vi "Tracker_Settings.vi"(0 "input cluster":T3, 2 "Directory Exists?":refnum<vi>) -> (1 "output cluster":T4)   [LabVIEW 2015]
uses:
  <vilib>/vision/Avi1.llb/AviRefnum.ctl
  <vilib>/userdefined/High Color/IMAQdx.ctl
panel:
  out "custom 2 timing array":dbl[](array[numeric])
  out "custom timing array":dbl[](array[numeric])
  out "puff timing array":dbl[](array[numeric])
  out "tap timing array":dbl[](array[numeric])
  out "AFG Settings":dbl[][](array[numeric])
  out "settings value cluster":T5
  out "Output  ROI Array":dbl[][](array[numeric])
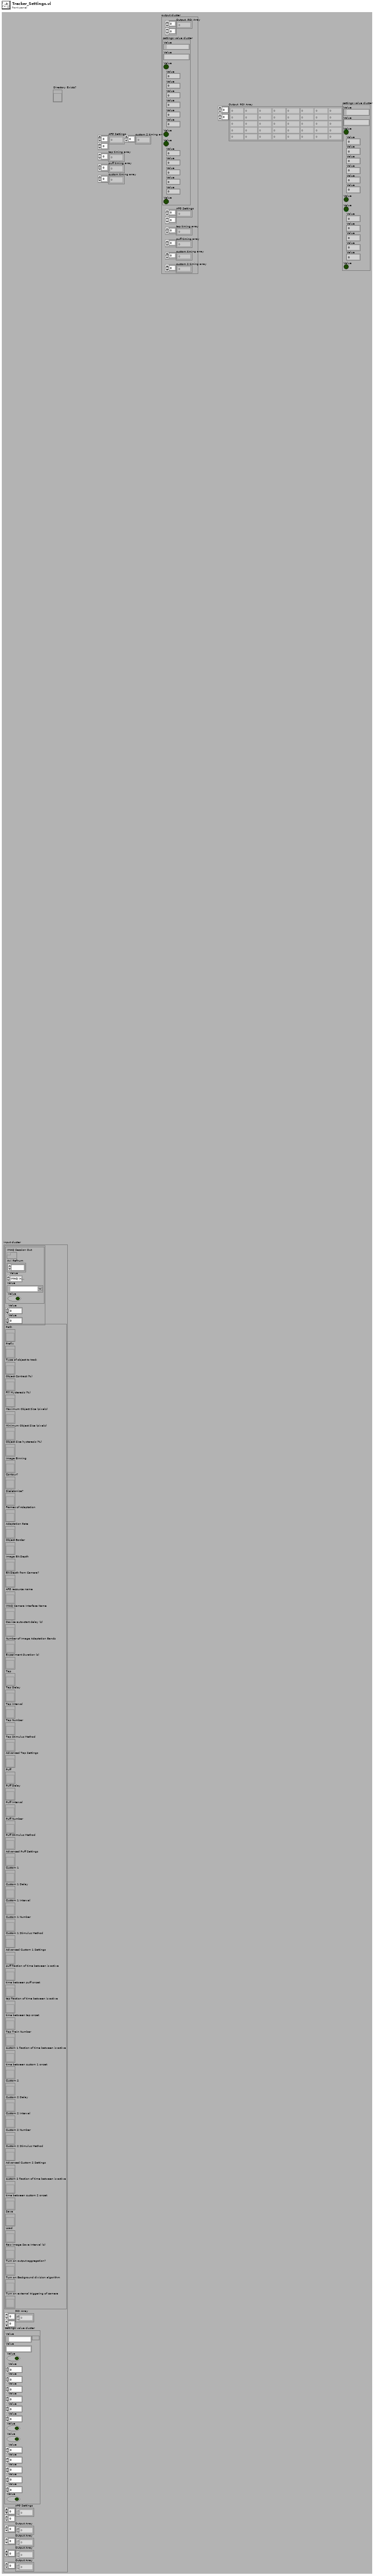
[diagram p1: front panel]
types:
  T1 = typedef "AviRefnum.ctl" = refnum<k1>
  T2 = typedef "IMAQdx.ctl" = refnum<k21>
  T3 = cluster{cluster{cluster{"IMAQ Session Out":refnum<k11>, "Avi Refnum":T1, "Value":enum32{"IMAQ interface", "IMAQdx interface", "AVI file"}, "Value":T2, "Value":bool}, "Value":i32, "Value":i32}, cluster{"Path":refnum<vi>, "Prefix":refnum<vi>, "Type of object to track":refnum<vi>, "Object Contrast (%)":refnum<vi>, "Fill Hysteresis (%)":refnum<vi>, "Maximum Object Size (pixels)":refnum<vi>, "Minimum Object Size (pixels)":refnum<vi>, "Object Size hysteresis (%)":refnum<vi>, "Image Binning":refnum<vi>, "Contour?":refnum<vi>, "Skeletonize?":refnum<vi>, "Frames of Adaptation":refnum<vi>, "Adaptation Rate":refnum<vi>, "Object Border":refnum<vi>, "Image Bit Depth":refnum<vi>, "Bit Depth from Camera?":refnum<vi>, "AFG resource name":refnum<vi>, "IMAQ Camera Interface Name":refnum<vi>, "Device auto-start delay (s)":refnum<vi>, "Number of Image Adaptation Bands":refnum<vi>, "Experiment Duration (s)":refnum<vi>, "Tap":refnum<vi>, "Tap Delay":refnum<vi>, "Tap Interval":refnum<vi>, "Tap Number":refnum<vi>, "Tap Stimulus Method":refnum<vi>, "Advanced Tap Settings":refnum<vi>, "Puff":refnum<vi>, "Puff Delay":refnum<vi>, "Puff Interval":refnum<vi>, "Puff Number":refnum<vi>, "Puff Stimulus Method":refnum<vi>, "Advanced Puff Settings":refnum<vi>, "Custom 1":refnum<vi>, "Custom 1 Delay":refnum<vi>, "Custom 1 Interval":refnum<vi>, "Custom 1 Number":refnum<vi>, "Custom 1 Stimulus Method":refnum<vi>, "Advanced Custom 1 Settings":refnum<vi>, "puff fraction of time between is active":refnum<vi>, "time between puff onset":refnum<vi>, "tap fraction of time between is active":refnum<vi>, "time between tap onset":refnum<vi>, "Tap Train Number":refnum<vi>, "custom 1 fraction of time between is active":refnum<vi>, "time between custom 1 onset":refnum<vi>, "Custom 2":refnum<vi>, "Custom 2 Delay":refnum<vi>, "Custom 2 Interval":refnum<vi>, "Custom 2 Number":refnum<vi>, "Custom 2 Stimulus Method":refnum<vi>, "Advanced Custom 2 Settings":refnum<vi>, "custom 2 fraction of time between is active":refnum<vi>, "time between custom 2 onset":refnum<vi>, "Save":refnum<vi>, "Load":refnum<vi>, "Raw Image Save Interval (s)":refnum<vi>, "Turn on output aggregation?":refnum<vi>, "Turn on Background division algorithm":refnum<vi>, "Turn on external triggering of camera":refnum<vi>}, "ROI Array":dbl[][], "settings value cluster":cluster{"Value":path, "Value":string, "Value":bool, "Value":dbl, "Value":dbl, "Value":i32, "Value":i32, "Value":dbl, "Value":u16, "Value":bool, "Value":bool, "Value":i32, "Value":i32, "Value":i32, "Value":u32, "Value":i32, "Value":bool}, "AFG Settings":dbl[][], "Output Array":dbl[], "Output Array":dbl[], "Output Array":dbl[], "Output Array":dbl[]}
  T4 = cluster{"Output  ROI Array":dbl[][], "settings value cluster":cluster{"Value":path, "Value":string, "Value":bool, "Value":dbl, "Value":dbl, "Value":i32, "Value":i32, "Value":dbl, "Value":u16, "Value":bool, "Value":bool, "Value":i32, "Value":i32, "Value":i32, "Value":u32, "Value":i32, "Value":bool}, "AFG Settings":dbl[][], "tap timing array":dbl[], "puff timing array":dbl[], "custom timing array":dbl[], "custom 2 timing array":dbl[]}
  T5 = cluster{"Value":path, "Value":string, "Value":bool, "Value":dbl, "Value":dbl, "Value":i32, "Value":i32, "Value":dbl, "Value":u16, "Value":bool, "Value":bool, "Value":i32, "Value":i32, "Value":i32, "Value":u32, "Value":i32, "Value":bool}
  T6 = cluster{cluster{"IMAQ Session Out":refnum<k11>, "Avi Refnum":T1, "Value":enum32{"IMAQ interface", "IMAQdx interface", "AVI file"}, "Value":T2, "Value":bool}, "Value":i32, "Value":i32}
  T7 = cluster{"Path":refnum<vi>, "Prefix":refnum<vi>, "Type of object to track":refnum<vi>, "Object Contrast (%)":refnum<vi>, "Fill Hysteresis (%)":refnum<vi>, "Maximum Object Size (pixels)":refnum<vi>, "Minimum Object Size (pixels)":refnum<vi>, "Object Size hysteresis (%)":refnum<vi>, "Image Binning":refnum<vi>, "Contour?":refnum<vi>, "Skeletonize?":refnum<vi>, "Frames of Adaptation":refnum<vi>, "Adaptation Rate":refnum<vi>, "Object Border":refnum<vi>, "Image Bit Depth":refnum<vi>, "Bit Depth from Camera?":refnum<vi>, "AFG resource name":refnum<vi>, "IMAQ Camera Interface Name":refnum<vi>, "Device auto-start delay (s)":refnum<vi>, "Number of Image Adaptation Bands":refnum<vi>, "Experiment Duration (s)":refnum<vi>, "Tap":refnum<vi>, "Tap Delay":refnum<vi>, "Tap Interval":refnum<vi>, "Tap Number":refnum<vi>, "Tap Stimulus Method":refnum<vi>, "Advanced Tap Settings":refnum<vi>, "Puff":refnum<vi>, "Puff Delay":refnum<vi>, "Puff Interval":refnum<vi>, "Puff Number":refnum<vi>, "Puff Stimulus Method":refnum<vi>, "Advanced Puff Settings":refnum<vi>, "Custom 1":refnum<vi>, "Custom 1 Delay":refnum<vi>, "Custom 1 Interval":refnum<vi>, "Custom 1 Number":refnum<vi>, "Custom 1 Stimulus Method":refnum<vi>, "Advanced Custom 1 Settings":refnum<vi>, "puff fraction of time between is active":refnum<vi>, "time between puff onset":refnum<vi>, "tap fraction of time between is active":refnum<vi>, "time between tap onset":refnum<vi>, "Tap Train Number":refnum<vi>, "custom 1 fraction of time between is active":refnum<vi>, "time between custom 1 onset":refnum<vi>, "Custom 2":refnum<vi>, "Custom 2 Delay":refnum<vi>, "Custom 2 Interval":refnum<vi>, "Custom 2 Number":refnum<vi>, "Custom 2 Stimulus Method":refnum<vi>, "Advanced Custom 2 Settings":refnum<vi>, "custom 2 fraction of time between is active":refnum<vi>, "time between custom 2 onset":refnum<vi>, "Save":refnum<vi>, "Load":refnum<vi>, "Raw Image Save Interval (s)":refnum<vi>, "Turn on output aggregation?":refnum<vi>, "Turn on Background division algorithm":refnum<vi>, "Turn on external triggering of camera":refnum<vi>}
  T8 = cluster{"IMAQ Session Out":refnum<k11>, "Avi Refnum":T1, "Value":enum32{"IMAQ interface", "IMAQdx interface", "AVI file"}, "Value":T2, "Value":bool}
  T9 = cluster{dbl[][], dbl[][], dbl[], dbl[], dbl[], dbl[]}
  T10 = cluster{cluster{"Path":refnum<vi>, "Prefix":refnum<vi>, "Type of object to track":refnum<vi>, "Object Contrast (%)":refnum<vi>, "Fill Hysteresis (%)":refnum<vi>, "Maximum Object Size (pixels)":refnum<vi>, "Minimum Object Size (pixels)":refnum<vi>, "Object Size hysteresis (%)":refnum<vi>, "Image Binning":refnum<vi>, "Contour?":refnum<vi>, "Skeletonize?":refnum<vi>, "Frames of Adaptation":refnum<vi>, "Adaptation Rate":refnum<vi>, "Object Border":refnum<vi>, "Image Bit Depth":refnum<vi>, "Bit Depth from Camera?":refnum<vi>, "AFG resource name":refnum<vi>, "IMAQ Camera Interface Name":refnum<vi>, "Device auto-start delay (s)":refnum<vi>, "Number of Image Adaptation Bands":refnum<vi>, "Experiment Duration (s)":refnum<vi>, "Tap":refnum<vi>, "Tap Delay":refnum<vi>, "Tap Interval":refnum<vi>, "Tap Number":refnum<vi>, "Tap Stimulus Method":refnum<vi>, "Advanced Tap Settings":refnum<vi>, "Puff":refnum<vi>, "Puff Delay":refnum<vi>, "Puff Interval":refnum<vi>, "Puff Number":refnum<vi>, "Puff Stimulus Method":refnum<vi>, "Advanced Puff Settings":refnum<vi>, "Custom 1":refnum<vi>, "Custom 1 Delay":refnum<vi>, "Custom 1 Interval":refnum<vi>, "Custom 1 Number":refnum<vi>, "Custom 1 Stimulus Method":refnum<vi>, "Advanced Custom 1 Settings":refnum<vi>, "puff fraction of time between is active":refnum<vi>, "time between puff onset":refnum<vi>, "tap fraction of time between is active":refnum<vi>, "time between tap onset":refnum<vi>, "Tap Train Number":refnum<vi>, "custom 1 fraction of time between is active":refnum<vi>, "time between custom 1 onset":refnum<vi>, "Custom 2":refnum<vi>, "Custom 2 Delay":refnum<vi>, "Custom 2 Interval":refnum<vi>, "Custom 2 Number":refnum<vi>, "Custom 2 Stimulus Method":refnum<vi>, "Advanced Custom 2 Settings":refnum<vi>, "custom 2 fraction of time between is active":refnum<vi>, "time between custom 2 onset":refnum<vi>, "Save":refnum<vi>, "Load":refnum<vi>, "Raw Image Save Interval (s)":refnum<vi>, "Turn on output aggregation?":refnum<vi>, "Turn on Background division algorithm":refnum<vi>, "Turn on external triggering of camera":refnum<vi>}, path, "ROI Array":dbl[][], "AFG Settings":dbl[][], "Output Array":dbl[], "Output Array":dbl[], "Output Array":dbl[], "Output Array":dbl[]}
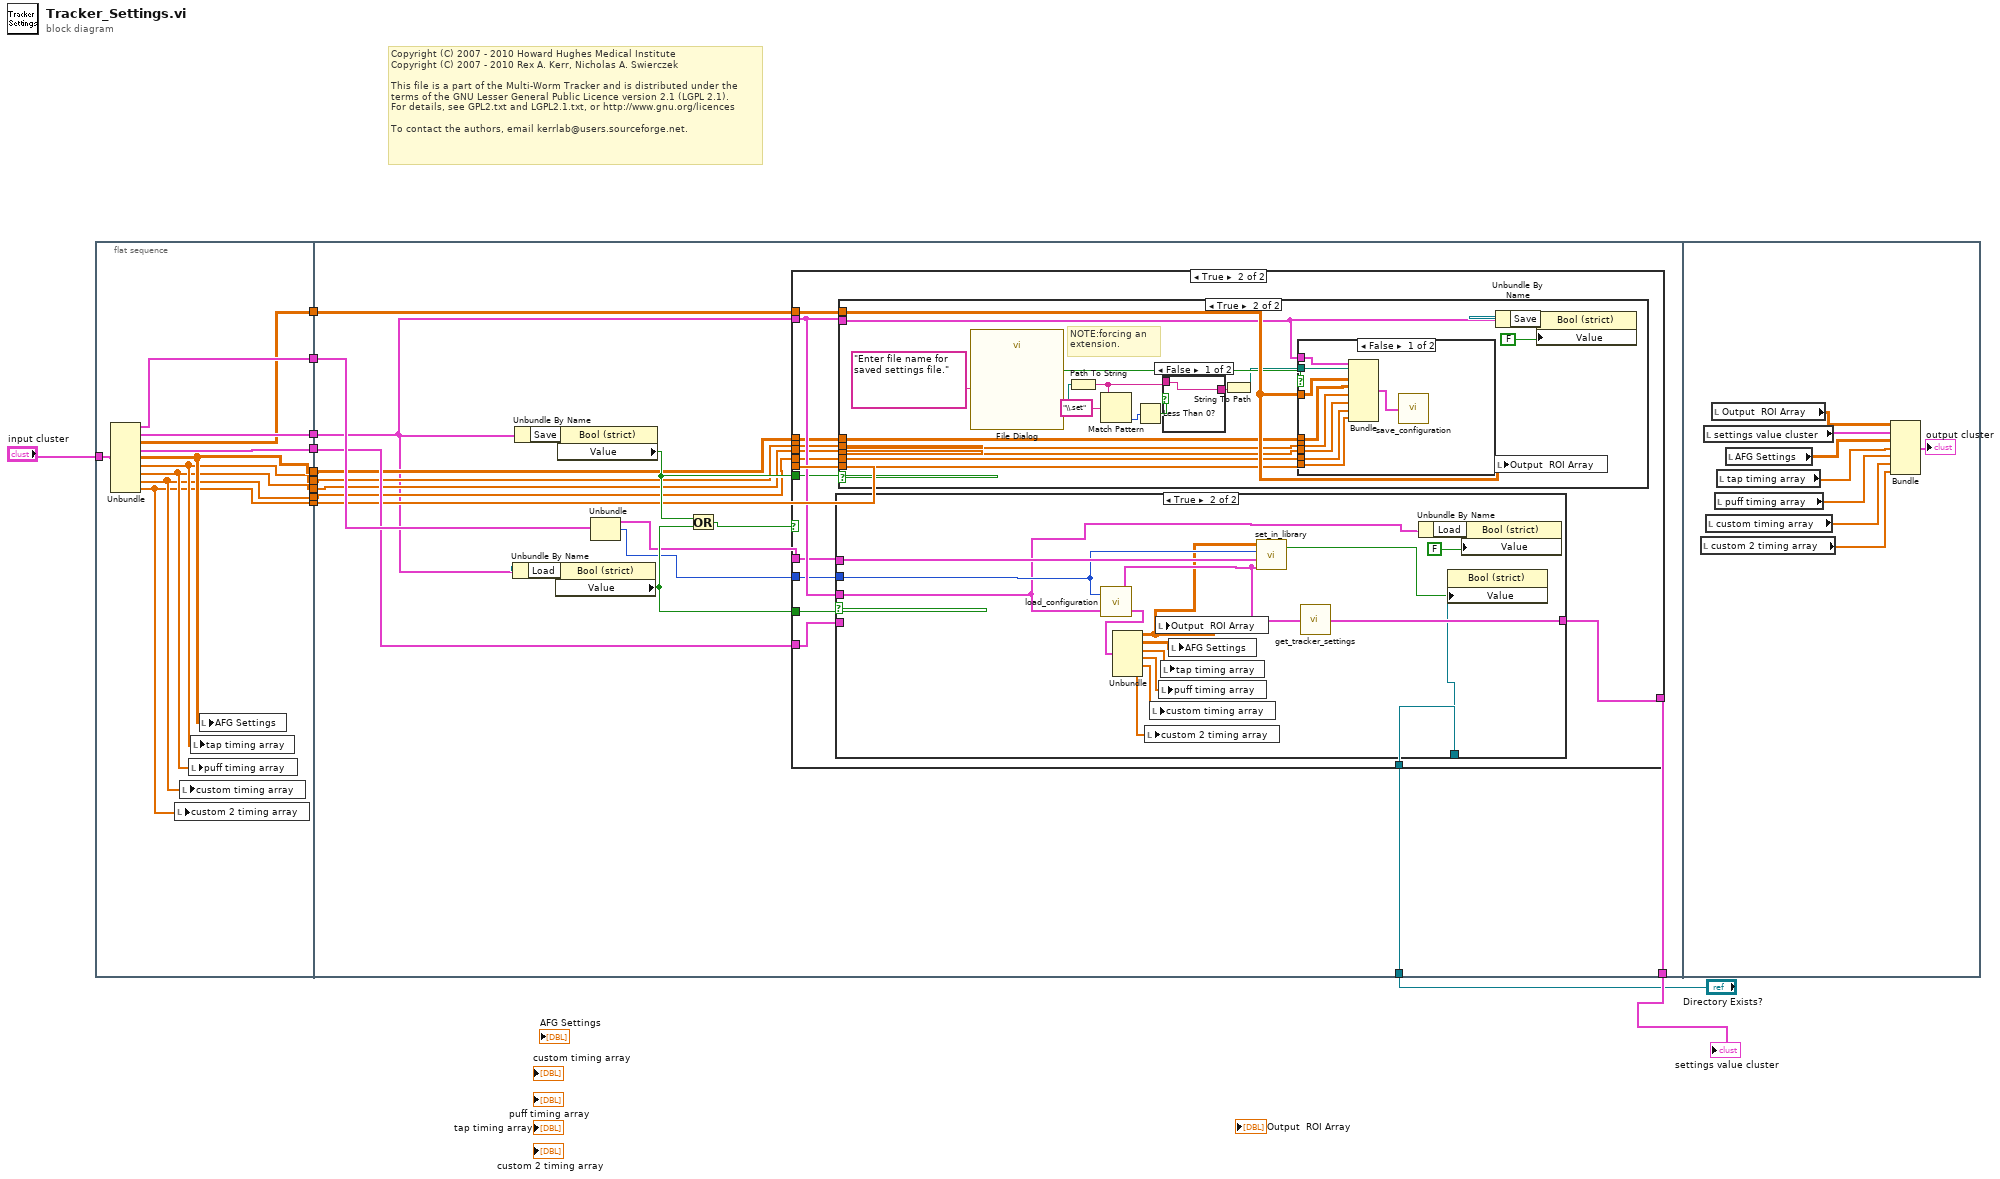
[diagram p0: block diagram]
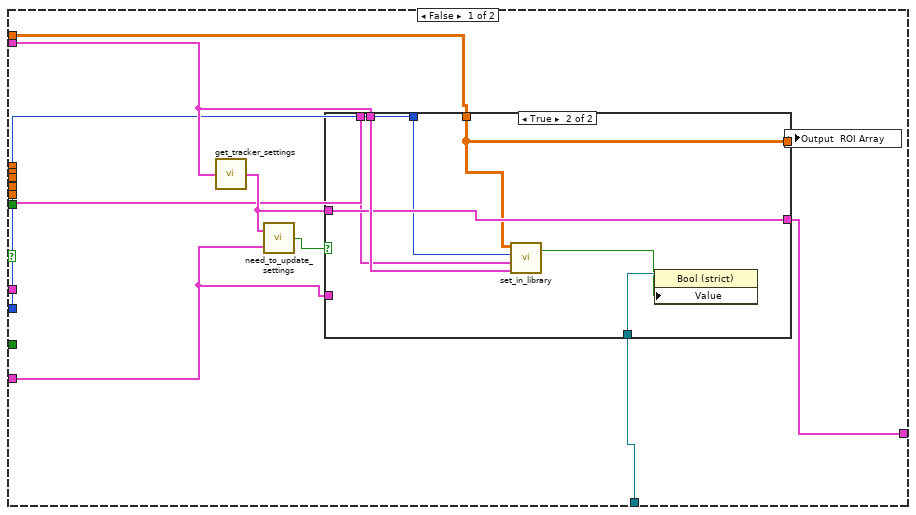
[diagram p2: hidden frame]
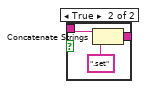
[diagram p6: hidden frame]
diagram:
  # "Copyright (C) 2007 - 2010 Howard Hughes Medical Institute\nCopyright (C) 2007 - 2010 Rex A. Kerr, Nicholas A. Swierczek\n \nThis file is a part of the Multi-Worm Tracker and is distributed under the\nterms of the GNU Lesser General Public Licence version 2.1 (LGPL 2.1).\nFor details, see GPL2.txt and LGPL2.1.txt, or http://www.gnu.org/licences\n \nTo contact the authors, email kerrlab@users.sourceforge.net."
  n1 = flat-sequence {
    tunnel: "input cluster" -> [w22]
    tunnel: [w13] -> w10
    tunnel: [w14] -> w9
    tunnel: [w15] -> w8
    tunnel: [w16] -> w7
    tunnel: [w17] -> w6
    tunnel: [w20] -> w5
    tunnel: [w21] -> w4
    tunnel: [w19] -> w3
    tunnel: [w18] -> w2
    tunnel: [w39] -> w12
    tunnel: "Directory Exists?" -> [w38]
    tunnel: w10 -> [w29]
    tunnel: w9 -> [w28]
    tunnel: w8 -> [w27]
    tunnel: w7 -> [w26]
    tunnel: w6 -> [w25]
    tunnel: w5 -> [w23]
    tunnel: w4 -> [w31]
    tunnel: w3 -> [w30]
    tunnel: w2 -> [w24]
    frame #0 {
      n2 = Unbundle(w22) -> (w21:T6, w20:T7, "ROI Array"=w18:dbl[][], "settings value cluster"=w19:T5, "AFG Settings"=w17:dbl[][], "Output Array"=w16:dbl[], "Output Array"=w15:dbl[], "Output Array"=w14:dbl[], "Output Array"=w13:dbl[])
      n3 = local write "custom 2 timing array"(w13) -> ()
      n4 = local write "custom timing array"(w14) -> ()
      n5 = local write "puff timing array"(w15) -> ()
      n6 = local write "tap timing array"(w16) -> ()
      n7 = local write "AFG Settings"(w17) -> ()
    }
    frame #1 {
      n8 = Unbundle By Name(w23) -> ("Load"=w35:refnum<vi>)
      n9 = Unbundle By Name(w23) -> ("Save"=w37:refnum<vi>)
      n10 = property class="Bool (strict)"(reference=w35) -> ("Value"=w34:bool)  [unwired: 1 in, 2 out]
      n11 = property class="Bool (strict)"(reference=w37) -> ("Value"=w36:bool)  [unwired: 1 in, 2 out]
      n12 = Unbundle(w31) -> (w32:T8, "Value"=w33:i32)  [unwired: 1 out]
      n13 = Or(x=w36, y=w34) -> (x .or. y?=w40:bool)
      n14 = case shown="True" w40 {
        tunnel: w23 -> [w49 w73]
        tunnel: w36 -> [_ w72]
        tunnel: w34 -> [_ w71]
        tunnel: w30 -> [w44 w70]
        tunnel: w33 -> [w48 w68]
        tunnel: [w46 w69] -> w39
        tunnel: w32 -> [w45 w67]
        tunnel: w24 -> [w43 w65]
        tunnel: w38 -> [w41 w66]
        tunnel: w25 -> [_ w64]
        tunnel: w26 -> [_ w63]
        tunnel: w27 -> [_ w62]
        tunnel: w28 -> [_ w61]
        tunnel: w29 -> [_ w60]
        frame False {
          n15 = call "get_tracker_settings.vi"("Cluster"=w49) -> ("settings value cluster"=w47:T5)
          n16 = call "need_to_update_settings.vi"("previous settings value cluster"=w44, "settings value cluster"=w47) -> ("New Settings Exist?"=w50:bool)
          n17 = case shown="True" w50 {
            tunnel: [w52 w58] -> w46
            tunnel: w49 -> [_ w59]
            tunnel: w48 -> [_ w56]
            tunnel: w44 -> [w52 _]
            tunnel: w47 -> [_ w58]
            tunnel: w45 -> [_ w57]
            tunnel: w43 -> [w51 w55]
            tunnel: [w51 w55] -> w42
            tunnel: w41 -> [_ w54]
            frame False {
            }
            frame True {
              n18 = call "set_in_library.vi"("Cluster"=w59, "camera cluster"=w57, "Tracker Handle"=w56, "Array"=w55) -> ("Directory Exists?"=w53:bool)  [unwired: 1 out]
              n19 = property class="Bool (strict)"(reference=w54, "Value"=w53) -> ()  [unwired: 1 in, 2 out]
            }
          }
          n20 = local write "Output  ROI Array"(w42) -> ()
        }
        frame True {
          n21 = case shown="True" w71 {
            tunnel: w73 -> [_ w84]
            tunnel: [w74 w89] -> w69
            tunnel: w70 -> [w74 _]
            tunnel: w68 -> [_ w87]
            tunnel: w67 -> [_ w88]
            tunnel: w66 -> [_ w83]
            frame False {
            }
            frame True {
              n22 = call "load_configuration.vi"("Cluster"=w84, "Handle"=w87) -> (0:"output cluster"=w81:T9, 1:"output cluster"=w90:T7)
              n23 = Unbundle(w81) -> (w80:dbl[][], w79:dbl[][], w78:dbl[], w77:dbl[], w76:dbl[], w75:dbl[])
              n24 = local write "custom 2 timing array"(w75) -> ()
              n25 = local write "custom timing array"(w76) -> ()
              n26 = local write "Output  ROI Array"(w80) -> ()
              n27 = local write "puff timing array"(w77) -> ()
              n28 = local write "tap timing array"(w78) -> ()
              n29 = local write "AFG Settings"(w79) -> ()
              n30 = call "set_in_library.vi"("Cluster"=w90, "camera cluster"=w88, "Tracker Handle"=w87, "Array"=w80) -> ("Directory Exists?"=w82:bool)  [unwired: 1 out]
              n31 = call "get_tracker_settings.vi"("Cluster"=w90) -> ("settings value cluster"=w89:T5)
              n32 = Unbundle By Name(w84) -> ("Load"=w86:refnum<vi>)
              n33 = property class="Bool (strict)"(reference=w83, "Value"=w82) -> ()  [unwired: 1 in, 2 out]
              n34 = property class="Bool (strict)"(reference=w86, "Value"=FALSE) -> ()  [unwired: 1 in, 2 out]
            }
          }
          n35 = case shown="True" w72 {
            tunnel: w73 -> [_ w105]
            tunnel: w65 -> [_ w108]
            tunnel: w64 -> [_ w102]
            tunnel: w63 -> [_ w101]
            tunnel: w62 -> [_ w100]
            tunnel: w61 -> [_ w99]
            tunnel: w60 -> [_ w98]
            frame False {
            }
            frame True {
              # "NOTE:forcing an \nextension."
              n36 = call "File Dialog"("prompt"="Enter file name for saved settings file.") -> ("selected path"=w95:path, "cancelled"=w103:bool)  [unwired: 11 in, 2 out]
              n37 = Path To String(path=w95) -> (string=w94:string)
              n38 = Match Pattern(string=w94, regular expression="\\.set") -> (offset past match=w93:i32)  [unwired: 1 in, 3 out]
              n39 = Less Than 0?(x=w93) -> (x < 0?=w92:bool)
              n40 = case shown="False" w92 {
                tunnel: [w109 w111] -> w96
                tunnel: w94 -> [w109 w110]
                frame False {
                }
                frame True {
                  n41 = Concatenate Strings(w110, ".set" ("name or relative path")) -> (w111:string)
                }
              }
              n42 = String To Path(string=w96) -> (path=w97:path)
              n43 = case shown="False" w103 {
                tunnel: w108 -> [w119 _]
                tunnel: w105 -> [w121 _]
                tunnel: w97 -> [w120 _]
                tunnel: w102 -> [w118 _]
                tunnel: w101 -> [w117 _]
                tunnel: w100 -> [w116 _]
                tunnel: w99 -> [w115 _]
                tunnel: w98 -> [w114 _]
                frame False {
                  n44 = Bundle(w121, w120, "ROI Array"=w119, "AFG Settings"=w118, "Output Array"=w117, "Output Array"=w116, "Output Array"=w115, "Output Array"=w114) -> (w113:T10)  [unwired: 1 in]
                  n45 = call "save_configuration.vi"("input cluster"=w113) -> ()
                }
                frame True {
                }
              }
              n46 = local write "Output  ROI Array"(w108) -> ()
              n47 = Unbundle By Name(w105) -> ("Save"=w107:refnum<vi>)
              n48 = property class="Bool (strict)"(reference=w107, "Value"=FALSE) -> ()  [unwired: 1 in, 2 out]
            }
          }
        }
      }
    }
    frame #2 {
      n49 = local read "custom 2 timing array"() -> (w123:dbl[])
      n50 = local read "settings value cluster"() -> (w128:T5)
      n51 = local read "custom timing array"() -> (w124:dbl[])
      n52 = local read "Output  ROI Array"() -> (w129:dbl[][])
      n53 = local read "puff timing array"() -> (w125:dbl[])
      n54 = local read "tap timing array"() -> (w126:dbl[])
      n55 = local read "AFG Settings"() -> (w127:dbl[][])
      n56 = Bundle("Output  ROI Array"=w129, "settings value cluster"=w128, "AFG Settings"=w127, "tap timing array"=w126, "puff timing array"=w125, "custom timing array"=w124, "custom 2 timing array"=w123) -> (→"output cluster":T4)  [unwired: 1 in]
    }
  }
  "settings value cluster" <- w12
